vi "peak_value_calculate_A_clean.vi"(0 "IO Module\\AI 1 Data N-1 2":i16, 1 "IO Module\\AI 1 Data N-2 3":i16, 2 "IO Module\\AI 1 Data N-2 2":i16, 3 "Boolean in":bool, 4 "IO Module\\AI 1 Data N-3 2":i16, 6 "IO Module\\AI 1 Data N 3":i16, 7 "IO Module\\AI 1 Data N":i16, 8 "IO Module\\AI 1 Data N-1 3":i16, 9 "IO Module\\AI 1 Data N-3":i16, 10 "IO Module\\AI 1 Data N 2":i16, 11 "IO Module\\AI 1 Data N-1":i16, 13 "IO Module\\AI 1 Data N-2":i16) -> (14 "bin_number":i16, 15 "Read Ready":bool, 16 "Spike Value":i16, 19 "first_row":bool)   [LabVIEW 2017]
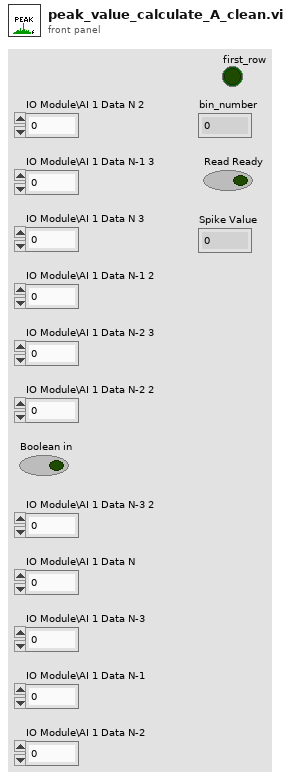
[diagram p1: front panel]
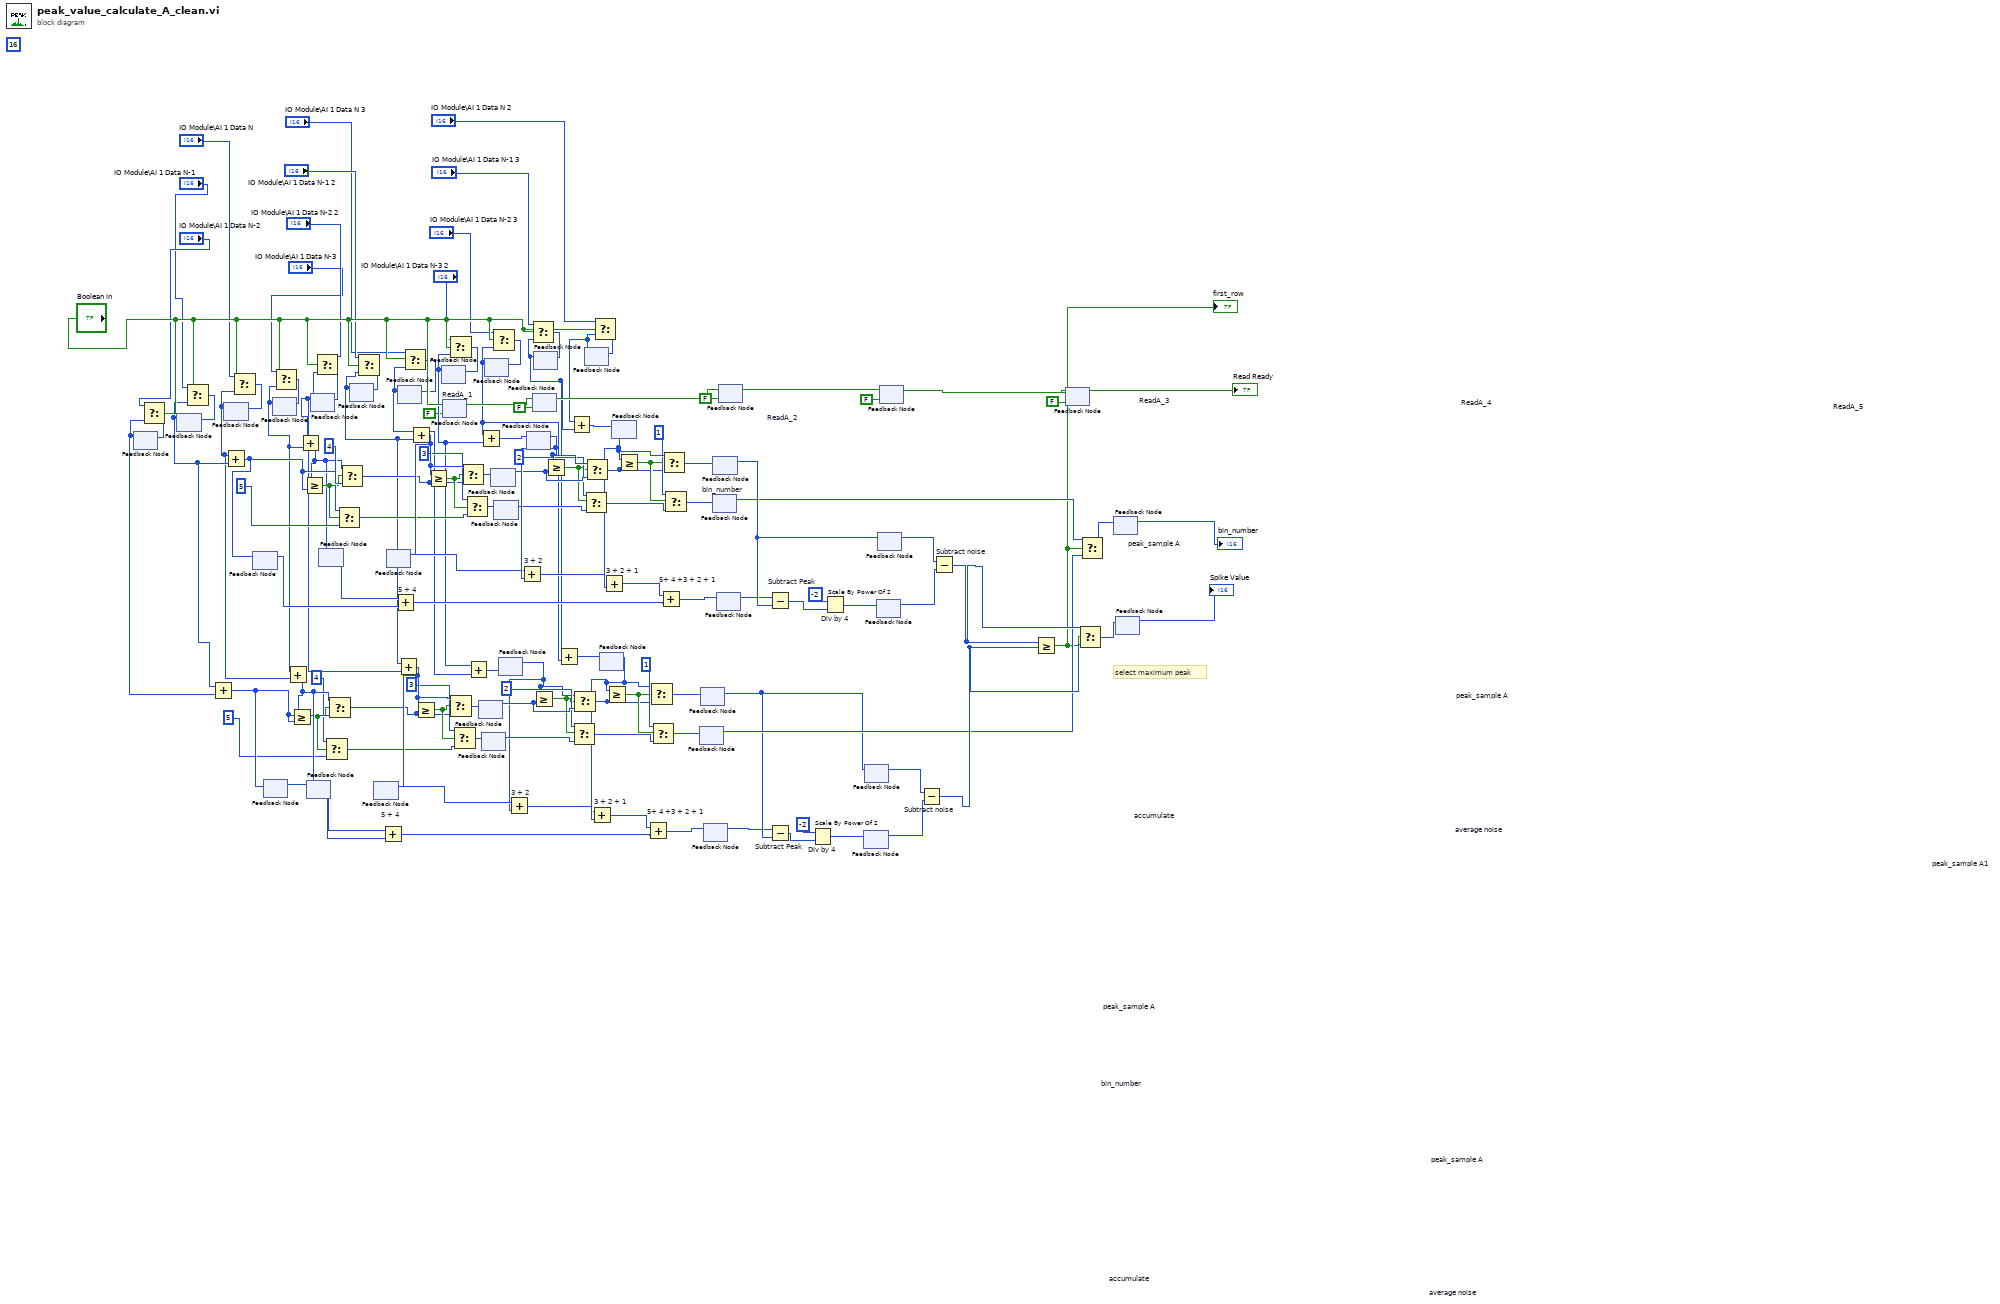
[diagram p0: block diagram]
diagram:
  (unwired) 16
  # "select maximum peak"
  n1 = feedback #1() -> (w65:i16)  [unwired: 1 in]
  n2 = Select(t="IO Module\\AI 1 Data N-2", s="Boolean in", f=w65) -> (s? t:f=w86:i16)
  n3 = feedback-in #1(w86) -> ()
  n4 = feedback #2() -> (w64:i16)  [unwired: 1 in]
  n5 = Select(t="IO Module\\AI 1 Data N-1", s="Boolean in", f=w64) -> (s? t:f=w75:i16)
  n6 = feedback-in #2(w75) -> ()
  n7 = Add(x=w64, y=w65) -> (x+y=w29:i16)
  n8 = feedback #3() -> (w63:i16)  [unwired: 1 in]
  n9 = Add(x=w63, y=w64) -> (x+y=w113:i16)
  n10 = Select(t="IO Module\\AI 1 Data N", s="Boolean in", f=w63) -> (s? t:f=w76:i16)
  n11 = feedback-in #3(w76) -> ()
  n12 = feedback #4() -> (w115:i16)  [unwired: 1 in]
  n13 = feedback-in #4(w113) -> ()
  n14 = feedback #5() -> (w32:i16)  [unwired: 1 in]
  n15 = feedback-in #5(w29) -> ()
  n16 = feedback #6() -> (w62:i16)  [unwired: 1 in]
  n17 = Select(t="IO Module\\AI 1 Data N-3", s="Boolean in", f=w62) -> (s? t:f=w88:i16)
  n18 = feedback-in #6(w88) -> ()
  n19 = Add(x=w62, y=w63) -> (x+y=w30:i16)
  n20 = Greater Or Equal?(x=w30, y=w29) -> (x >= y?=w9:bool)
  n21 = feedback #7() -> (w33:i16)  [unwired: 1 in]
  n22 = feedback-in #7(w30) -> ()
  n23 = feedback #8() -> (w61:i16)  [unwired: 1 in]
  n24 = Add(x=w61, y=w62) -> (x+y=w50:i16)
  n25 = Greater Or Equal?(x=w50, y=w113) -> (x >= y?=w89:bool)
  n26 = Select(t="IO Module\\AI 1 Data N-2 2", s="Boolean in", f=w61) -> (s? t:f=w82:i16)
  n27 = feedback-in #8(w82) -> ()
  n28 = feedback #9() -> (w116:i16)  [unwired: 1 in]
  n29 = feedback-in #9(w50) -> ()
  n30 = Select(t=i16 4 ("count"), s=w9, f=i16 5 ("count")) -> (s? t:f=w15:i16)
  n31 = Select(t=w30, s=w9, f=w29) -> (s? t:f=w12:i16)
  n32 = Select(t=i16 4 ("count"), s=w89, f=i16 5 ("count")) -> (s? t:f=w95:i16)
  n33 = Select(t=w50, s=w89, f=w113) -> (s? t:f=w92:i16)
  n34 = feedback #10() -> (w60:i16)  [unwired: 1 in]
  n35 = Select(t="IO Module\\AI 1 Data N-1 2", s="Boolean in", f=w60) -> (s? t:f=w83:i16)
  n36 = feedback-in #10(w83) -> ()
  n37 = feedback #11() -> (w34:i16)  [unwired: 1 in]
  n38 = Add "5 + 4"(x=w33, y=w32) -> (x+y=w37:i16)
  n39 = feedback #12() -> (w117:i16)  [unwired: 1 in]
  n40 = Add "5 + 4"(x=w116, y=w115) -> (x+y=w122:i16)
  n41 = Add(x=w60, y=w61) -> (x+y=w31:i16)
  n42 = feedback-in #11(w31) -> ()
  n43 = feedback #13() -> (w59:i16)  [unwired: 1 in]
  n44 = Select(t="IO Module\\AI 1 Data N 3", s="Boolean in", f=w59) -> (s? t:f=w84:i16)
  n45 = feedback-in #13(w84) -> ()
  n46 = Add(x=w59, y=w60) -> (x+y=w114:i16)
  n47 = feedback-in #12(w114) -> ()
  n48 = Greater Or Equal?(x=w31, y=w12) -> (x >= y?=w13:bool)
  n49 = Greater Or Equal?(x=w114, y=w92) -> (x >= y?=w93:bool)
  n50 = feedback #14() -> (w58:i16)  [unwired: 1 in]
  n51 = feedback #15 "ReadA_1"(FALSE ("Boolean in")) -> (w111:bool)
  n52 = feedback-in #15("Boolean in") -> ()
  n53 = Select(t="IO Module\\AI 1 Data N-3 2", s="Boolean in", f=w58) -> (s? t:f=w70:i16)
  n54 = feedback-in #14(w70) -> ()
  n55 = Select(t=w31, s=w13, f=w12) -> (s? t:f=w16:i16)
  n56 = Select(t=i16 3 ("count"), s=w13, f=w15) -> (s? t:f=w20:i16)
  n57 = Select(t=w114, s=w93, f=w92) -> (s? t:f=w96:i16)
  n58 = Select(t=i16 3 ("count"), s=w93, f=w95) -> (s? t:f=w100:i16)
  n59 = Add(x=w58, y=w59) -> (x+y=w17:i16)
  n60 = feedback #16() -> (w27:i16)  [unwired: 1 in]
  n61 = feedback-in #16(w16) -> ()
  n62 = feedback #17() -> (w28:i16)  [unwired: 1 in]
  n63 = feedback-in #17(w20) -> ()
  n64 = feedback #18() -> (w57:i16)  [unwired: 1 in]
  n65 = Add(x=w57, y=w58) -> (x+y=w97:i16)
  n66 = feedback #19() -> (w108:i16)  [unwired: 1 in]
  n67 = feedback-in #19(w96) -> ()
  n68 = Select(t="IO Module\\AI 1 Data N-2 3", s="Boolean in", f=w57) -> (s? t:f=w68:i16)
  n69 = feedback-in #18(w68) -> ()
  n70 = feedback #20() -> (w109:i16)  [unwired: 1 in]
  n71 = feedback-in #20(w100) -> ()
  n72 = feedback #21() -> (w1:i16)  [unwired: 1 in]
  n73 = feedback-in #21(w17) -> ()
  n74 = Add "3 + 2"(x=w34, y=w1) -> (x+y=w35:i16)
  n75 = feedback #22() -> (w118:i16)  [unwired: 1 in]
  n76 = Add "3 + 2"(x=w117, y=w118) -> (x+y=w120:i16)
  n77 = feedback-in #22(w97) -> ()
  n78 = Greater Or Equal?(x=w1, y=w27) -> (x >= y?=w18:bool)
  n79 = feedback #23 "ReadA_2"(FALSE ("Boolean in")) -> (w112:bool)
  n80 = feedback-in #23(w111) -> ()
  n81 = feedback #24() -> (w56:i16)  [unwired: 1 in]
  n82 = Select(t="IO Module\\AI 1 Data N-1 3", s="Boolean in", f=w56) -> (s? t:f=w66:i16)
  n83 = feedback-in #24(w66) -> ()
  n84 = Greater Or Equal?(x=w118, y=w108) -> (x >= y?=w98:bool)
  n85 = Add(x=w56, y=w57) -> (x+y=w8:i16)
  n86 = Select(t=i16 2 ("count"), s=w18, f=w28) -> (s? t:f=w23:i16)
  n87 = Select(t=w1, s=w18, f=w27) -> (s? t:f=w21:i16)
  n88 = feedback #25() -> (w87:i16)  [unwired: 1 in]
  n89 = Add(x=w87, y=w56) -> (x+y=w101:i16)
  n90 = Select(t=i16 2 ("count"), s=w98, f=w109) -> (s? t:f=w104:i16)
  n91 = Select(t=w118, s=w98, f=w108) -> (s? t:f=w102:i16)
  n92 = Select(t="IO Module\\AI 1 Data N 2", s="Boolean in", f=w87) -> (s? t:f=w78:i16)
  n93 = feedback-in #25(w78) -> ()
  n94 = feedback #26() -> (w7:i16)  [unwired: 1 in]
  n95 = Add "3 + 2 + 1"(x=w7, y=w35) -> (x+y=w36:i16)
  n96 = feedback-in #26(w8) -> ()
  n97 = Greater Or Equal?(x=w7, y=w21) -> (x >= y?=w22:bool)
  n98 = feedback #27() -> (w119:i16)  [unwired: 1 in]
  n99 = Add "3 + 2 + 1"(x=w119, y=w120) -> (x+y=w121:i16)
  n100 = feedback-in #27(w101) -> ()
  n101 = Greater Or Equal?(x=w119, y=w102) -> (x >= y?=w103:bool)
  n102 = Add "5+ 4 +3 + 2 + 1"(x=w36, y=w37) -> (x+y=w38:i16)
  n103 = Select(t=w7, s=w22, f=w21) -> (s? t:f=w25:i16)
  n104 = Select(t=i16 1 ("count"), s=w22, f=w23) -> (s? t:f=w26:i16)
  n105 = Add "5+ 4 +3 + 2 + 1"(x=w121, y=w122) -> (x+y=w123:i16)
  n106 = Select(t=w119, s=w103, f=w102) -> (s? t:f=w106:i16)
  n107 = Select(t=i16 1 ("count"), s=w103, f=w104) -> (s? t:f=w107:i16)
  n108 = feedback #28 "bin_number"() -> (w52:i16)  [unwired: 1 in]
  n109 = feedback-in #28(w26) -> ()
  n110 = feedback #29 "peak_sample A"() -> (w43:i16)  [unwired: 1 in]
  n111 = feedback-in #29(w25) -> ()
  n112 = feedback #30 "accumulate"() -> (w39:i16)  [unwired: 1 in]
  n113 = feedback-in #30(w38) -> ()
  n114 = feedback #31 "bin_number"() -> (w51:i16)  [unwired: 1 in]
  n115 = feedback-in #31(w107) -> ()
  n116 = feedback #32 "peak_sample A"() -> (w128:i16)  [unwired: 1 in]
  n117 = feedback-in #32(w106) -> ()
  n118 = feedback #33 "accumulate"() -> (w124:i16)  [unwired: 1 in]
  n119 = feedback-in #33(w123) -> ()
  n120 = feedback #34 "ReadA_3"(FALSE ("Boolean in")) -> (w129:bool)
  n121 = feedback-in #34(w112) -> ()
  n122 = Subtract "Subtract Peak"(x=w124, y=w128) -> (x-y=w125:i16)
  n123 = Subtract "Subtract Peak"(x=w39, y=w43) -> (x-y=w40:i16)
  n124 = Scale By Power Of 2 "Div by 4"(n=i16 -2, x=w40) -> (x*2^n=w42:i16)
  n125 = Scale By Power Of 2 "Div by 4"(n=i16 -2, x=w125) -> (x*2^n=w127:i16)
  n126 = feedback #35 "average noise"() -> (w45:i16)  [unwired: 1 in]
  n127 = feedback-in #35(w42) -> ()
  n128 = feedback #36 "peak_sample A"() -> (w44:i16)  [unwired: 1 in]
  n129 = feedback-in #36(w43) -> ()
  n130 = feedback #37 "average noise"() -> (w131:i16)  [unwired: 1 in]
  n131 = feedback-in #37(w127) -> ()
  n132 = feedback #38 "peak_sample A"() -> (w130:i16)  [unwired: 1 in]
  n133 = feedback-in #38(w128) -> ()
  n134 = feedback #39 "ReadA_4"(FALSE ("Boolean in")) -> (w132:bool)
  n135 = feedback-in #39(w129) -> ()
  n136 = Subtract "Subtract noise"(x=w44, y=w45) -> (x-y=w53:i16)
  n137 = Subtract "Subtract noise"(x=w130, y=w131) -> (x-y=w54:i16)
  n138 = Greater Or Equal?(x=w54, y=w53) -> (x >= y?=w47:bool)
  "first_row" <- w47
  n139 = feedback #40 "ReadA_5"(FALSE ("Boolean in")) -> (→"Read Ready":bool)
  n140 = feedback-in #40(w132) -> ()
  n141 = Select(t=w54, s=w47, f=w53) -> (s? t:f=w48:i16)
  n142 = Select(t=w51, s=w47, f=w52) -> (s? t:f=w46:i16)
  n143 = feedback #41 ("peak_sample A1")() -> (→"bin_number":i16)  [unwired: 1 in]
  n144 = feedback-in #41(w46) -> ()
  n145 = feedback #42 "peak_sample A1"() -> (→"Spike Value":i16)  [unwired: 1 in]
  n146 = feedback-in #42(w48) -> ()
